vi "Reading Calibration Data.vi"(10 "output cluster":T1) -> (3 "Error":bool)   [LabVIEW 2015]
uses:
  Controls/Cal Refs.ctl
  Miscellaneous/Globals.vi
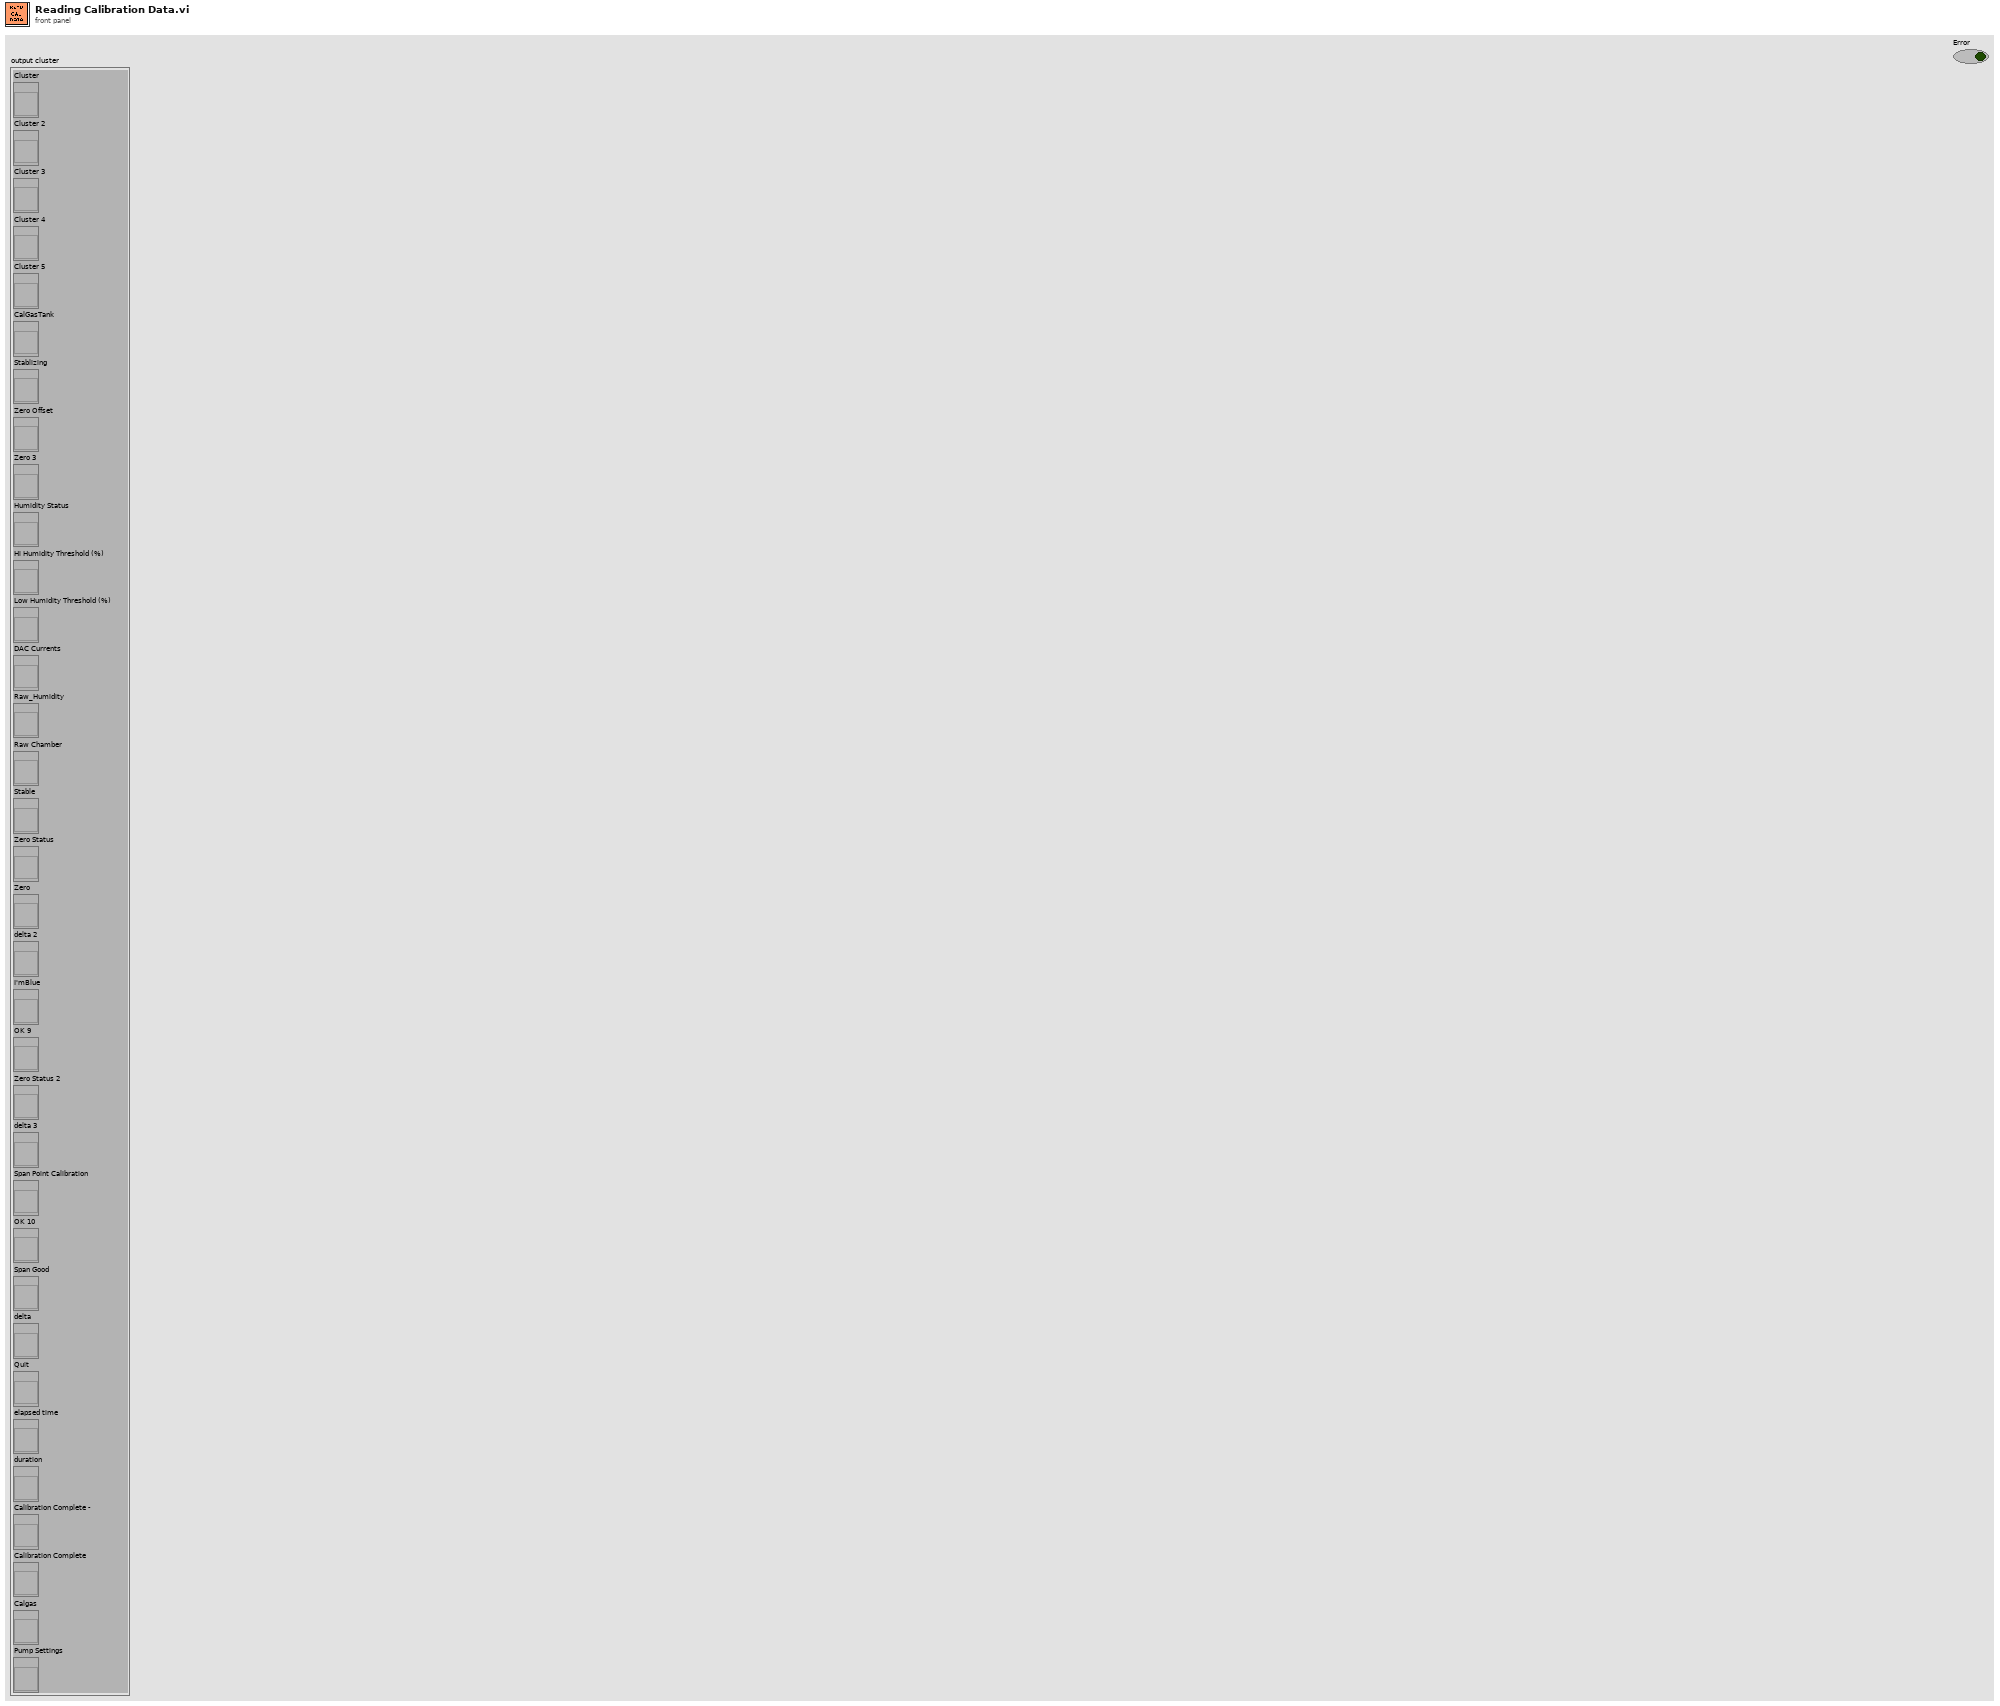
[diagram p1: front panel]
types:
  T1 = typedef "Cal Refs.ctl" = cluster{"Cluster":refnum<vi>, "Cluster 2":refnum<vi>, "Cluster 3":refnum<vi>, "Cluster 4":refnum<vi>, "Cluster 5":refnum<vi>, "CalGasTank":refnum<vi>, "Stablizing":refnum<vi>, "Zero Offset":refnum<vi>, "Zero 3":refnum<vi>, "Humidity Status":refnum<vi>, "Hi Humidity Threshold (%)":refnum<vi>, "Low Humidity Threshold (%)":refnum<vi>, "DAC Currents":refnum<vi>, "Raw_Humidity":refnum<vi>, "Raw Chamber":refnum<vi>, "Stable":refnum<vi>, "Zero Status":refnum<vi>, "Zero":refnum<vi>, "delta 2":refnum<vi>, "I'mBlue":refnum<vi>, "OK 9":refnum<vi>, "Zero Status 2":refnum<vi>, "delta 3":refnum<vi>, "Span Point Calibration":refnum<vi>, "OK 10":refnum<vi>, "Span Good":refnum<vi>, "delta":refnum<vi>, "Quit":refnum<vi>, "elapsed time":refnum<vi>, "duration":refnum<vi>, "Calibration Complete -":refnum<vi>, "Calibration Complete":refnum<vi>, "Calgas":refnum<vi>, "Pump Settings":refnum<vi>}
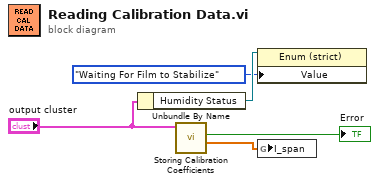
[diagram p0: block diagram]
diagram:
  n1 = Unbundle By Name("output cluster") -> ("Humidity Status"=w5:refnum<vi>)
  n2 = call "Storing Calibration Coefficients.vi"("output cluster"="output cluster") -> ("Array"=w2:dbl[], "Error"=→"Error":bool)  [unwired: 9 in]
  n3 = property class="Enum (strict)"(reference=w5, "Value"=enum16{"Waiting For Film to Stabilize"}."Waiting For Film to Stabilize" ("Enum")) -> ()  [unwired: 1 in, 2 out]
  n4 = global write "Globals.vi" "I_span"(w2) -> ()
